vi "EditContact.vi"(7 "LabVIEW Web Service Request":refnum<class "Web Request.lvclass">) -> ()   [LabVIEW 2014]
doc: "This HTTP Method VI accepts a contact as form post data and either updates an existing contact or inserts a new one into the address book data store. It then redirects back to the contact list."
uses:
  <vilib>/wsapi/Web Request.lvclass
  Libraries/Contact Data/Command.ctl
  Libraries/Contact Data/Contact Data.lvlib
panel:
  # "Because this is an HTTP Method VI, LabVIEW Web Service Request is populated automatically."
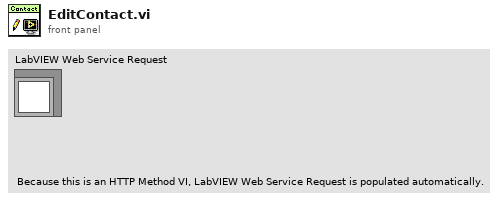
[diagram p1: front panel]
types:
  T1 = typedef "Contact Data.lvlib/Command.ctl" = enum16{"Set All Contacts", "Load", "Save", "Get All Data", "Get Single Data (ID)", "Get Single Data", "Set Position", "Set Destinations", "Set Controls", "Remove Single Data", "Remove UUID Contact", "Set Single ALL", "Is Data Modified", "Import Data"}
  T2 = typedef "Contact Data.lvlib/Contact.ctl" = cluster{"ID":u32, "UUID":string, "Name":string, "Iteration":i32, "Posit Array":T3[], "Controls":T4, "DestArray":T5[], "SetSpeed":dbl, "Speed":dbl}
  T3 = typedef "Contact Data.lvlib/Position.ctl" = cluster{"X":dbl, "Y":dbl, "Z":dbl}
  T4 = typedef "Contact Data.lvlib/Controls.ctl" = cluster{"throttle":dbl, "brake":dbl, "horn":dbl, "wait":dbl}
  T5 = typedef "Contact Data.lvlib/DestinationCluster.ctl" = cluster{"Desination":string, "DestControls":T6, "Timer":u32, "Set Timer":u32, "Time Stamp":timestamp, "Repeat?":bool, "Optional Data":string, "Distance":dbl}
  T6 = typedef "Contact Data.lvlib/DesinationControls.ctl" = enum16{"Tracker", "Manual", "Stop", "Station DateTime", "Station Timer", "Maintain"}
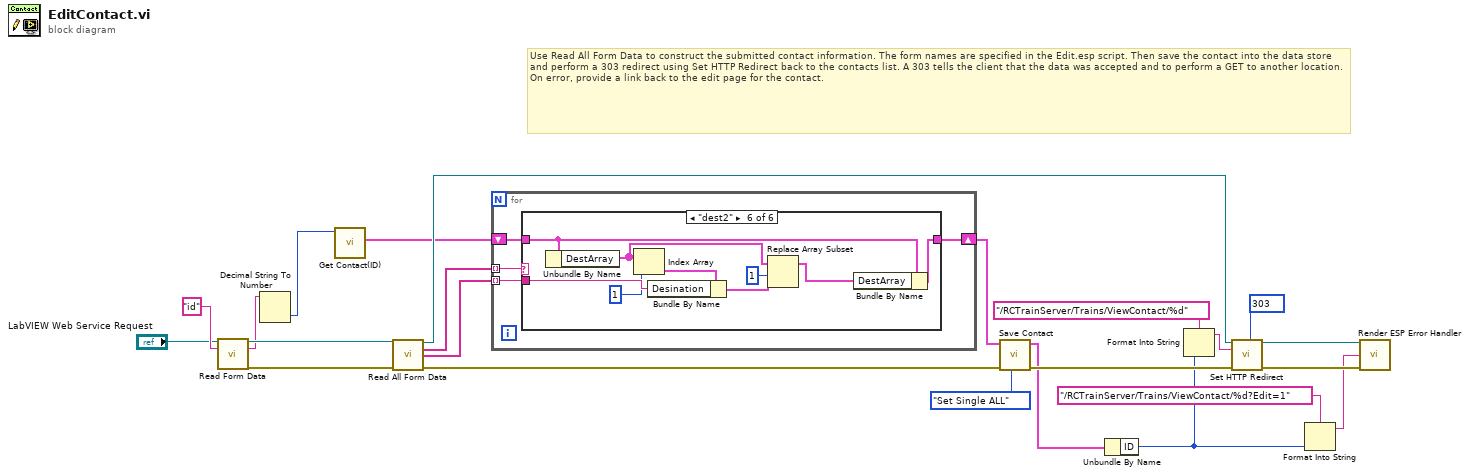
[diagram p0: block diagram]
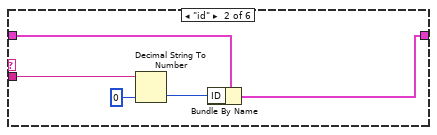
[diagram p3: hidden frame]
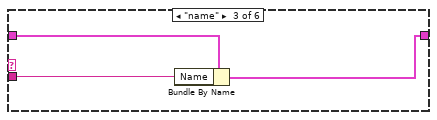
[diagram p4: hidden frame]
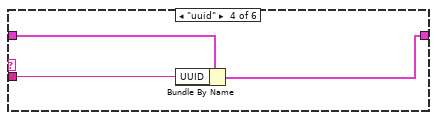
[diagram p5: hidden frame]
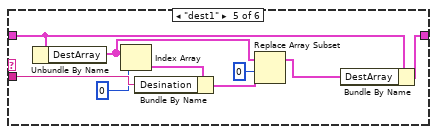
[diagram p6: hidden frame]
diagram:
  w23 = 303 items=["100"=100, "101"=101, "200"=200, "201"=201, "202"=202, "203"=203, "204"=204, "205"=205, "206"=206, "300"=300, "301"=301, "302"=302, "303"=303, "304"=304, "305"=305, "306"=306, "307"=307, "400"=400, "401"=401, "402"=402, "403"=403, "404"=404, "405"=405, "406"=406, "407"=407, "408"=408, "409"=409, "410"=410, "411"=411, "412"=412, "413"=413, "414"=414, "415"=415, "416"=416, "417"=417, "500"=500, "501"=501, "502"=502, "503"=503, "504"=504, "505"=505] ("response code (307)")
  # "Use Read All Form Data to construct the submitted contact information. The form names are specified in the Edit.esp script. Then save the contact into the data store and perform a 303 redirect using Set HTTP Redirect back to the contacts list. A 303 tells the client that the data was accepted and to perform a GET to another location. On error, provide a link back to the edit page for the contact."
  n1 = call <vilib>:"Read Form Data.vi"("LabVIEW Web Service Request"="LabVIEW Web Service Request", "key"="id") -> ("LabVIEW Web Service Request out"=w9:refnum<class "Web Request.lvclass">, "value"=w7:string, "error out"=w8:errorcluster)  [unwired: 10 in, 1 out]
  n2 = Decimal String To Number(string=w7) -> (number=w6:i32)  [unwired: 2 in, 1 out]
  n3 = call "Get Contact(ID).vi"("ID"=w6) -> ("Contact"=w5:T2)  [unwired: 8 in, 2 out]
  n4 = call <vilib>:"Read All Form Data.vi"("LabVIEW Web Service Request"=w9, "error in (no error)"=w8) -> ("LabVIEW Web Service Request out"=w19:refnum<class "Web Request.lvclass">, "Key"=w21:string[], "Value"=w20:string[], "error out"=w18:errorcluster)  [unwired: 9 in, 1 out]
  n5 = for {
    tunnel: w21 -> [w27] mode=indexing
    tunnel: w20 -> [w26] mode=indexing
    shift-right: [w24] -> w15
    shift-left: w5 -> [w25]
    n6 = case shown="\"dest2\"" w27 {
      tunnel: w26 -> [_ w31 w34 w38 w45 w54]
      tunnel: w25 -> [w28 w33 w36 w39 w47 w56]
      tunnel: [w28 w32 w35 w37 w48 w57] -> w24
      frame Default {
      }
      frame "id" {
        n7 = Decimal String To Number(string=w31, default (0L)=u32 0 ("default (0 I32)")) -> (number=w30:u32)  [unwired: 1 in, 1 out]
        n8 = Bundle By Name(cluster=w33, "ID"=w30) -> (w32:T2)
      }
      frame "name" {
        n9 = Bundle By Name(cluster=w36, "Name"=w34) -> (w35:T2)
      }
      frame "uuid" {
        n10 = Bundle By Name(cluster=w39, "UUID"=w38) -> (w37:T2)
      }
      frame "dest1" {
        n11 = Unbundle By Name(w47) -> ("DestArray"=w43:T5[])
        n12 = Index Array(array=w43, index=0) -> (element=w46:T5)
        n13 = Bundle By Name(cluster=w46, "Desination"=w45) -> (w41:T5)
        n14 = Replace Array Subset(array=w43, new element=w41, index=0) -> (w40:T5[])
        n15 = Bundle By Name(cluster=w47, "DestArray"=w40) -> (w48:T2)
      }
      frame "dest2" {
        n16 = Unbundle By Name(w56) -> ("DestArray"=w52:T5[])
        n17 = Index Array(array=w52, index=1) -> (element=w55:T5)
        n18 = Bundle By Name(cluster=w55, "Desination"=w54) -> (w50:T5)
        n19 = Replace Array Subset(array=w52, new element=w50, index=1) -> (w49:T5[])
        n20 = Bundle By Name(cluster=w56, "DestArray"=w49) -> (w57:T2)
      }
    }
  }
  n21 = call "Save Contact.vi"("Command"=Command."Set Single ALL", "error in (no error)"=w18, "Contact"=w15) -> ("error out"=w17:errorcluster, "dup Contact"=w16:T2)  [unwired: 7 in]
  n22 = Unbundle By Name(w16) -> ("ID"=w3:u32)
  n23 = Format Into String(format string="/RCTrainServer/Trains/ViewContact/%d" ("redirect URL"), w3) -> (resulting string=w1:string)  [unwired: 2 in, 1 out]
  n24 = call <vilib>:"Set HTTP Redirect.vi"("LabVIEW Web Service Request"=w19, "redirect URL"=w1, "response code (307)"=w23, "error in (no error)"=w17) -> ("LabVIEW Web Service Request out"=w14:refnum<class "Web Request.lvclass">, "error out"=w13:errorcluster)  [unwired: 10 in]
  n25 = Format Into String(format string="/RCTrainServer/Trains/ViewContact/%d?Edit=1" ("Link"), w3) -> (resulting string=w12:string)  [unwired: 2 in, 1 out]
  n26 = call "Render ESP Error Handler.vi"("LabVIEW Web Service Request"=w14, "Link"=w12, "error in (no error)"=w13) -> ()  [unwired: 11 in, 2 out]
